vi "Keithley DMM6500 DAQ6500 Series Scanning Temperature With Thermocouples.vi"() -> ()   [LabVIEW 2019]
doc: "This example shows how to scan temperature with thermocouples"
uses:
  Public/Configure/Configure Temperature (Thermocouple).vi
  Public/Data/Read (Multiple Points).vi
  Keithley DMM6500 DAQ6500 Series.lvlib
panel:
  in  "Save Data?":bool
  in  "Buffer Element2 ()":i32(ring) items=["", "Date", "Extra", "Formatted", "Fractional", "Reading", "Relative", "Seconds", "Status", "Time", "Tstamp", "Unit", "CHAN", "Extra Form", "Extra Unit"]
  in  "Buffer Element1 ()":i32(ring) items=["", "Date", "Extra", "Formatted", "Fractional", "Reading", "Relative", "Seconds", "Status", "Time", "Tstamp", "Unit", "CHAN", "Extra Format", "Extra Unit"]
  in  "File Name(\"/usb1/scan24hr.csv\")":string="/usb1/scan24hr.csv"
  out "Measurements":dbl[](array[numeric])
  in  "Reference Junction Type (1: Internal)":i32(ring)=1 items=["Simulated", "Internal", "External"]
  in  "Thermocouple Type (3: K)":i32(ring)=3 items=["B", "E", "J", "K", "N", "R", "S", "T"]
  in  "Unit (1: Celsius)":i32(ring)=1 items=["Kelvin", "Celsius", "Fahrenheit"]
  in  "Reading Buffer Size (14400)":u32=14400
  in  "Reading Buffer (\"defbuffer1\")":string="defbuffer1"
  in  "Scan Interval (60 s)":dbl=60.0
  in  "Scan Count (1440)":u32=1440
  in  "Channel List (\"101:110\")":string="101:110"
  in  "VISA resource name":refnum<visa-resource-name>
  # "(c) 2018 National Instruments.  ALL RIGHTS RESERVED."
  # "This example VI demonstrates how to use the DAQ6500 Series to log thermocouple-based temperature\nmeasurement scans using internal cold-junction compensation (CJC) correction over a 24-hour period."
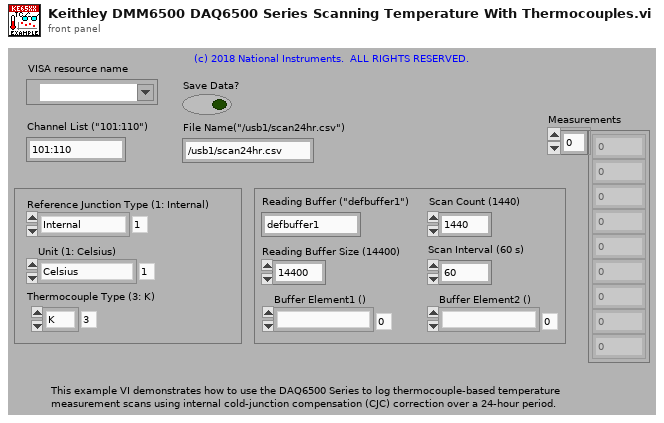
[diagram p1: front panel]
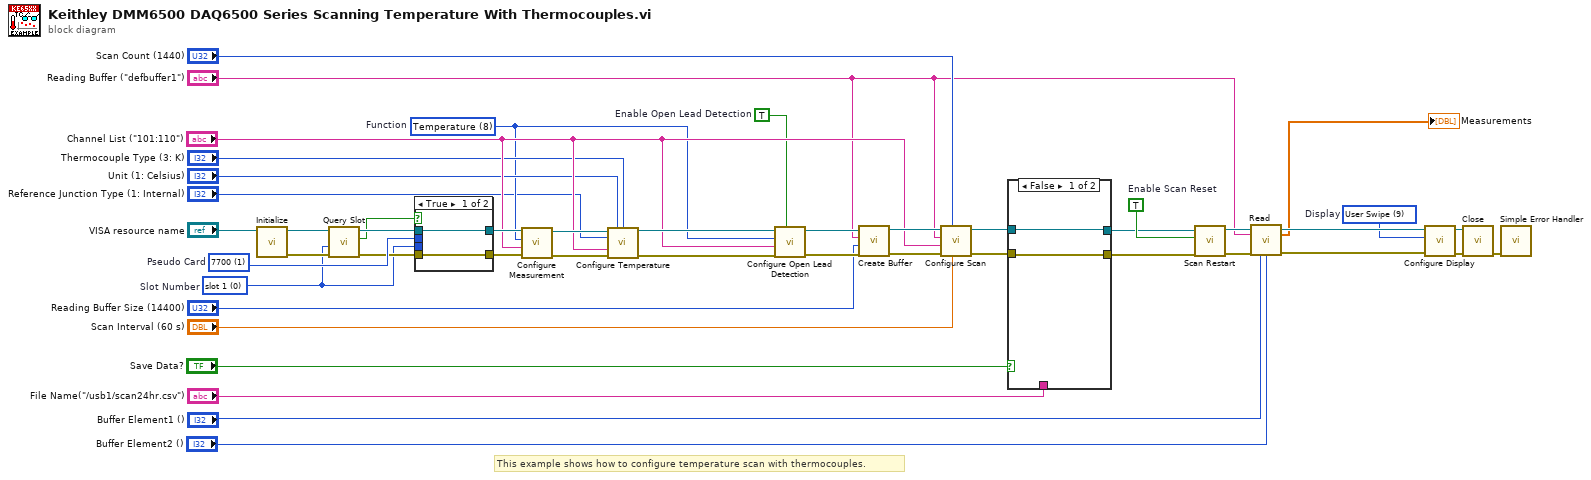
[diagram p0: block diagram]
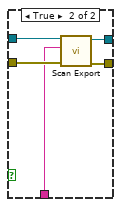
[diagram p2: hidden frame]
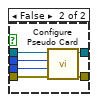
[diagram p3: hidden frame]
diagram:
  w17 = 9 items=["Home Screen", "Home with Large Readings", "Reading Table", "Graph", "Functions Swipe", "Graph Swipe", "Secondary Swipe", "Setting Swipe", "Statistic Swipe", "User Swipe", "Channel Swipe", "Nonswich Swipe", "Scan Swipe", "Control Channel", "Settings Channel", "Scan Channel"]  # Display
  w13 = 0 items=["slot 1", "slot 2"]  # Slot Number
  w33 = 1 items=["0", "7700", "7701", "7702", "7703", "7705", "7706", "7707", "7708", "7709", "7710", "7711", "7712"]  # Pseudo Card
  w20 = 8 items=[" Voltage DC", "Voltage AC", "Current DC", "Current AC", "Resistance", "4-wire Resistance", "Diode", "Capacitance", "Temperature", "Continuity", "Frequency", "Period", "Voltage Ratio", "Digitize Voltage", "Digitize Current"]  # Function
  w41 = TRUE  # Enable Scan Reset
  w21 = TRUE  # Enable Open Lead Detection
  # "This example shows how to configure temperature scan with thermocouples."
  n1 = call "Initialize.vi"("VISA resource name"="VISA resource name") -> ("error out"=w15:errorcluster, "VISA resource name out"=w44:refnum<visa-resource-name>)  [unwired: 9 in]
  n2 = call "Query Slot.vi"("error in (no error)"=w15, "Slot Number(0: slot 1)"=w13, "VISA resource name"=w44) -> ("error out"=w14:errorcluster, "Real Card In Slot"=w12:bool, "VISA resource name out"=w16:refnum<visa-resource-name>)  [unwired: 6 in]
  n3 = case shown="True" w12 {
    tunnel: [w48 w54] -> w43
    tunnel: [w47 w53] -> w42
    tunnel: w33 -> [_ w52]
    tunnel: w16 -> [w48 w51]
    tunnel: w14 -> [w47 w50]
    tunnel: w13 -> [_ w49]
    frame True {
    }
    frame False {
      n4 = call "Configure Pseudo Card.vi"("error in (no error)"=w50, "Slot Number (0: slot1)"=w49, "Pseudo Card (0:No pseudocard)"=w52, "VISA resource name"=w51) -> ("error out"=w53:errorcluster, "VISA resource name out"=w54:refnum<visa-resource-name>)  [unwired: 6 in]
    }
  }
  n5 = call "Configure Measurement.vi"("error in (no error)"=w42, "Channel List(\"\")"="Channel List (\"101:110\")", "Function (0: Voltage DC)"=w20, "VISA resource name"=w43) -> ("error out"=w30:errorcluster, "VISA resource name out"=w32:refnum<visa-resource-name>)  [unwired: 6 in]
  n6 = call-poly "Configure Temperature.vi"("VISA resource name"=w32, "Unit (1: Celsius)"="Unit (1: Celsius)", "Thermocouple Type (3: K)"="Thermocouple Type (3: K)", "Reference Junction Type (1: Internal)"="Reference Junction Type (1: Internal)", "Channel List(\"\")"="Channel List (\"101:110\")", "error in (no error)"=w30) -> ("VISA resource name out"=w31:refnum<visa-resource-name>, "error out"=w29:errorcluster)  [unwired: 8 in]
  n7 = call "Configure Open Lead Detection.vi"("Enable Open Lead Detection (F: Disable)"=w21, "error in (no error)"=w29, "Channel List(\"\")"="Channel List (\"101:110\")", "Function (5: 4-wire resistance)"=w20, "VISA resource name"=w31) -> ("error out"=w35:errorcluster, "VISA resource name out"=w36:refnum<visa-resource-name>)  [unwired: 5 in]
  n8 = call "Create Buffer.vi"("error in (no error)"=w35, "Buffer Size (10)"="Reading Buffer Size (14400)", "Buffer Name (\"\")"="Reading Buffer (\"defbuffer1\")", "VISA resource name"=w36) -> ("error out"=w37:errorcluster, "VISA resource name out"=w38:refnum<visa-resource-name>)  [unwired: 6 in]
  n9 = call "Configure Scan.vi"("Delay Seconds (0 s)"="Scan Interval (60 s)", "Scan Count (1)"="Scan Count (1440)", "error in (no error)"=w37, "Channel List(\"\")"="Channel List (\"101:110\")", "Reading Buffer (\"\")"="Reading Buffer (\"defbuffer1\")", "VISA resource name"=w38) -> ("error out"=w7:errorcluster, "VISA resource name out"=w8:refnum<visa-resource-name>)  [unwired: 4 in]
  n10 = case shown="False" "Save Data?" {
    tunnel: w8 -> [w56 w61]
    tunnel: w7 -> [w55 w60]
    tunnel: [w55 w59] -> w6
    tunnel: [w56 w58] -> w5
    tunnel: "File Name(\"/usb1/scan24hr.csv\")" -> [_ w57]
    frame False {
    }
    frame True {
      n11 = call "Scan Export.vi"("error in (no error)"=w60, "File Name (\"\")"=w57, "VISA resource name"=w61) -> ("error out"=w59:errorcluster, "VISA resource name out"=w58:refnum<visa-resource-name>)  [unwired: 7 in]
    }
  }
  n12 = call "Scan Restart.vi"("error in (no error)"=w6, "Enable Scan Reset (T: Enable)"=w41, "VISA resource name"=w5) -> ("error out"=w24:errorcluster, "VISA resource name out"=w25:refnum<visa-resource-name>)  [unwired: 7 in]
  n13 = call-poly "Read.vi"("VISA resource name"=w25, "Buffer Name (\"\")"="Reading Buffer (\"defbuffer1\")", "error in (no error)"=w24, "Buffer Element1 ()"="Buffer Element1 ()", "Buffer Element2 ()"="Buffer Element2 ()") -> ("VISA resource name out"=w23:refnum<visa-resource-name>, "Measurements"=→"Measurements":dbl[], "error out"=w10:errorcluster)  [unwired: 8 in]
  n14 = call "Configure Display.vi"("error in (no error)"=w10, "Display (0: Home Screen)"=w17, "VISA resource name"=w23) -> ("error out"=w9:errorcluster, "VISA resource name out"=w18:refnum<visa-resource-name>)  [unwired: 7 in]
  n15 = call "Close.vi"("error in (no error)"=w9, "VISA resource name"=w18) -> ("error out"=w46:errorcluster)  [unwired: 9 in]
  n16 = call <vilib>:"Simple Error Handler.vi"("error in (no error)"=w46) -> ()  [unwired: 4 in, 5 out]
